vi "libssh2_sftp_rmdir_ex.vi"(8 "error in (no error)":errorcluster, 10 "path":string, 11 "sftp":T1) -> (0 "error out":errorcluster)   [LabVIEW 2013, in "libssh2.lvlib"]
doc: "Remove a directory."
uses:
  libssh2.lvlib
  SFTP Refnum.ctl
  Not An SFTP Refnum.vi
  <vilib>/Utility/error.llb/Error Cluster From Error Code.vi
  Global Settings.vi
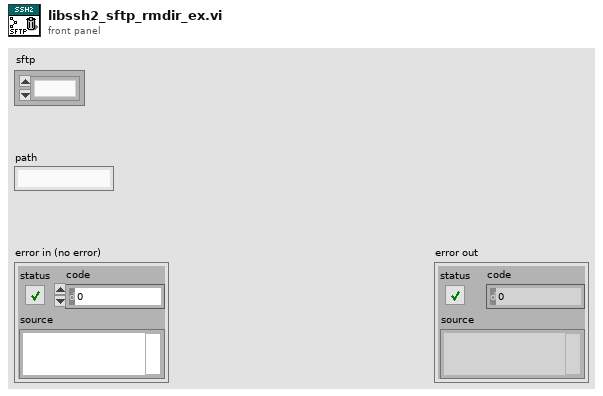
[diagram p1: front panel]
types:
  T1 = typedef "libssh2.lvlib/SFTP Refnum.ctl" = refnum<k1>
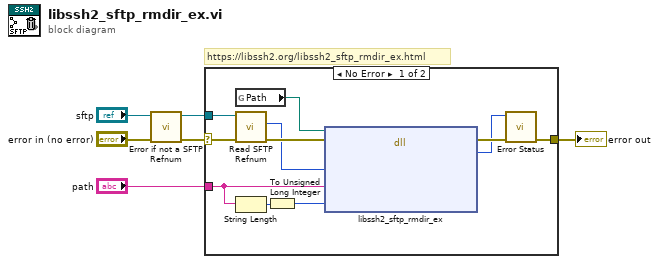
[diagram p0: block diagram]
diagram:
  # "https://libssh2.org/libssh2_sftp_rmdir_ex.html"
  n1 = call "Error if not a SFTP Refnum.vi"("error in (no error)"="error in (no error)", "sftp"="sftp") -> ("error out"=w5:errorcluster, "sftp out"=w4:T1)  [unwired: 8 in]
  n2 = case shown="No Error" w5 {
    selector: w5 -> [w16 w18]
    tunnel: w4 -> [w15 _]
    tunnel: [w11 w18] -> w3
    tunnel: "path" -> [w9 _]
    frame No Error {
      n3 = global read "Global Settings.vi" "Path"() -> (w17:path)
      n4 = call "Read SFTP Refnum.vi"("error in (no error)"=w16, "sftp"=w15) -> ("error out"=w14:errorcluster, "LIBSSH2_SFTP*"=w13:u64)  [unwired: 8 in]
      n5 = String Length(string=w9) -> (length=w8:i32)
      n6 = To Unsigned Long Integer(number=w8) -> (unsigned 32bit integer=w7:u32)
      n7 = dll-call lib="?" fn="libssh2_sftp_rmdir_ex"(path in=w17, error in=w14, "sftp"=w13, "path"=w9, "path_len"=w7) -> (error out=w12:errorcluster, "return value"=w10:i32)  [unwired: 4 in, 1 out]
      n8 = call "Error Status.vi"("error in (no error)"=w12, "return value"=w10) -> ("error out"=w11:errorcluster)  [unwired: 8 in, 1 out]
    }
    frame Error {
    }
  }
  "error out" <- w3
